vi "3.11-Get Half of Graph.vi"(1 "Start Turn":dbl, 2 "Magnitude":dbl, 3 "Angle":dbl) -> (0 "Array":dbl[](array[numeric]))   [LabVIEW 2011]
uses:
  3.0-Global.vi
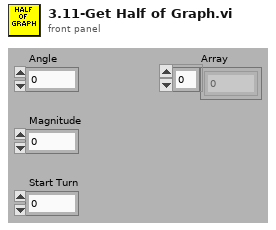
[diagram p1: front panel]
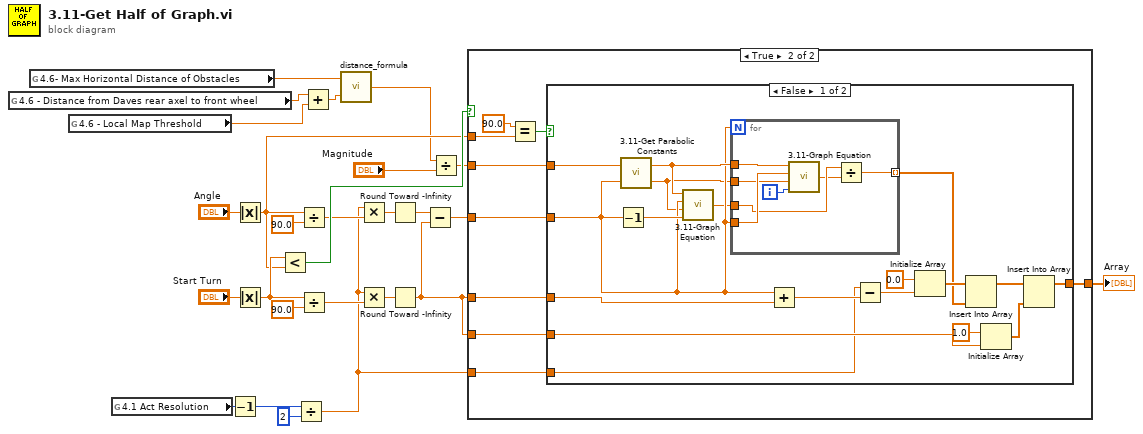
[diagram p0: block diagram]
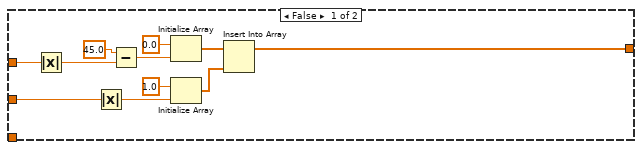
[diagram p2: hidden frame]
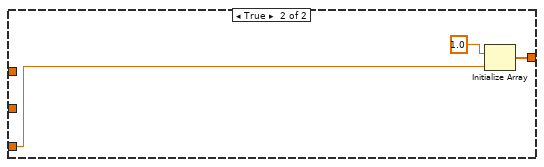
[diagram p3: hidden frame]
diagram:
  n1 = global read "3.0-Global.vi" "4.6 - Distance from Daves rear axel to front wheel"() -> (w2:dbl)
  n2 = global read "3.0-Global.vi" "4.6- Max Horizontal Distance of Obstacles"() -> (w5:dbl)
  n3 = global read "3.0-Global.vi" "4.6 - Local Map Threshold"() -> (w1:dbl)
  n4 = global read "3.0-Global.vi" "4.1 Act Resolution"() -> (w9:u32)
  n5 = Decrement(x=w9) -> (x-1=w7:u32)
  n6 = Absolute Value(x="Angle") -> (abs(x)=w10:dbl)
  n7 = Absolute Value(x="Start Turn") -> (abs(x)=w11:dbl)
  n8 = Less?(x=w11, y=w10) -> (x < y?=w18:bool)
  n9 = Divide(x=w7, y=u32 2) -> (x/y=w6:dbl)
  n10 = Divide(x=w10, y=90.0) -> (x/y=w15:dbl)
  n11 = Divide(x=w11, y=90.0) -> (x/y=w20:dbl)
  n12 = Add(x=w2, y=w1) -> (x+y=w4:dbl)
  n13 = call "distance_formula.vi"("X2 - X1"=w4, "Y2 - Y1"=w5) -> ("Distance"=w3:dbl)
  n14 = Multiply(x=w6, y=w15) -> (x*y=w12:dbl)
  n15 = Multiply(x=w6, y=w20) -> (x*y=w21:dbl)
  n16 = Round Toward -Infinity(1:w12) -> (0:w25:dbl)
  n17 = Round Toward -Infinity(1:w21) -> (0:w24:dbl)
  n18 = Subtract(x=w25, y=w24) -> (x-y=w23:dbl)
  n19 = Divide(x=w3, y="Magnitude") -> (x/y=w14:dbl)
  n20 = case shown="True" w18 {
    tunnel: w14 -> [_ w46]
    tunnel: [w35 w44] -> w26
    tunnel: w23 -> [_ w41]
    tunnel: w24 -> [w36 w45]
    tunnel: w24 -> [w32 w43]
    tunnel: w10 -> [_ w39]
    tunnel: w6 -> [_ w38]
    frame False {
      n21 = Absolute Value(x=w32) -> (abs(x)=w29:dbl)
      n22 = Absolute Value(x=w36) -> (abs(x)=w30:dbl)
      n23 = Subtract(x=45.0, y=w29) -> (x-y=w31:dbl)
      n24 = Initialize Array(0.0 ("element"), w31) -> (w28:dbl[])
      n25 = Initialize Array(1.0 ("element"), w30) -> (w27:dbl[])
      n26 = Insert Into Array(array=w28, new element=w27) -> (w35:dbl[])  [unwired: 1 in]
    }
    frame True {
      n27 = Equal?(x=90.0, y=w39) -> (x = y?=w42:bool)
      n28 = case shown="False" w42 {
        tunnel: w46 -> [w64 _]
        tunnel: w45 -> [w62 _]
        tunnel: [w61 w73] -> w44
        tunnel: w43 -> [w60 _]
        tunnel: w41 -> [w54 _]
        tunnel: w38 -> [w47 w72]
        frame False {
          n29 = Decrement(x=w54) -> (x-1=w56:dbl)
          n30 = call "3.11-Get Parabolic Constants.vi"("Number of affected points (z)"=w54, "Scaled Magnitude"=w64) -> ("Graph scale factor (b)"=w53:dbl, "parabolic constant (c)"=w55:dbl)
          n31 = call "3.11-Graph Equation.vi"("X"=w56, "Graph scale factor (b)"=w53, "Where it hits 0 (z)"=w54, "parabolic constant (c)"=w55) -> ("Y"=w52:dbl)
          n32 = for {
            N: w54 -> [_]
            tunnel: w55 -> [w68]
            tunnel: w53 -> [w69]
            tunnel: w54 -> [w71]
            tunnel: [w65] -> w48 mode=indexing
            tunnel: w52 -> [w67]
            i -> [w70]
            n33 = call "3.11-Graph Equation.vi"("X"=w70, "Graph scale factor (b)"=w69, "Where it hits 0 (z)"=w71, "parabolic constant (c)"=w68) -> ("Y"=w66:dbl)
            n34 = Divide(x=w67, y=w66) -> (x/y=w65:dbl)
          }
          n35 = Add(x=w54, y=w60) -> (x+y=w58:dbl)
          n36 = Subtract(x=w47, y=w58) -> (x-y=w57:dbl)
          n37 = Initialize Array(0.0 ("element"), w57) -> (w49:dbl[])
          n38 = Insert Into Array(array=w49, new element=w48) -> (w51:dbl[])  [unwired: 1 in]
          n39 = Initialize Array(1.0 ("element"), w62) -> (w50:dbl[])
          n40 = Insert Into Array(array=w51, new element=w50) -> (w61:dbl[])  [unwired: 1 in]
        }
        frame True {
          n41 = Initialize Array(1.0 ("element"), w72) -> (w73:dbl[])
        }
      }
    }
  }
  "Array" <- w26
